vi "ControlTimerValues (1).vi"() -> (3 "Array":i64[](array[numeric]))   [LabVIEW 2017]
uses:
  ControlTimersGLOBAL.vi
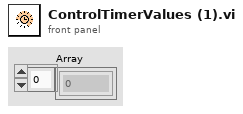
[diagram p1: front panel]
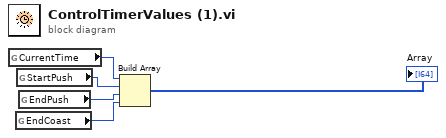
[diagram p0: block diagram]
diagram:
  n1 = global read "ControlTimersGLOBAL.vi" "CurrentTime"() -> (w1:i64)
  n2 = global read "ControlTimersGLOBAL.vi" "EndCoast"() -> (w4:i64)
  n3 = global read "ControlTimersGLOBAL.vi" "StartPush"() -> (w2:i64)
  n4 = global read "ControlTimersGLOBAL.vi" "EndPush"() -> (w3:i64)
  n5 = Build Array(w1, w2, w3, w4) -> (→"Array":i64[])
